vi "Calculate Bit Error Ratio.vi"(0 "in DFE mode?":bool, 5 "positive counts":T1, 7 "negative counts":T1, 11 "error in":errorcluster) -> (4 "bit error ratio":dbl, 6 "sample count":u64, 8 "error count":u64, 15 "error out":errorcluster)   [LabVIEW 2015, in "niHighSpeedSerial Eye Scan Single Point v1 Host.lvclass"]
doc: "Calculates the Bit Error Rate.\nWhen in LPM mode, the BER rate is computed as the (error count + 1)/(sample count)\nWhen in DFE mode, the BER rate is computed by taking the average of the positive BER and negative BER.\n\n<B>Input Parameters</B>\n\n<B>in DFE mode?</B> is true if Eye Scan is configured for DFE Equalization Mode.\n\n<B>positive counts</B> contains the positive UT sign sample and error counts when using DFE Equalization Mode.\nWhen using LPM Equalization Mode, contains the sample and error counts.\n\n<B>positive counts.sample count</B> is the positive sample count when using DFE mode, or the entire sample count when using LPM mode.\n\n<B>positive counts.error count</B> is the positive error count when using DFE mode, or the entire error count when using LPM mode.\n\n<B>negative counts</B> contains the negative UT sign sample and error counts when using DFE Equalization Mode.\nWhen using LPM Equalization Mode, 'negative counts' is unused.\n\n<B>negative counts.sample count</B> is the negative sample count when using DFE mode, or unused when using LPM mode.\n\n<B>negative counts.error count</B> is the negative error count when using DFE mode, or unused when using LPM mode.\n\n<B>error in</B> describes error conditions that occur before this node runs. This input provides standard 'error in' functionality.\n\n<B>Output Parameters</B>\n\n<B>bit error rate</B> is the calculated statistical bit error rate based on the number of error counts and sample counts received.\n\n<B>sample count</B> is the number of samples that have been measured on this point.\n\n<B>error count</B> is the number of errors that have been measured on this point.\n\n<B>error out</B> contains error information. This output provides standard 'error out' functionality."
uses:
  <instrlib>/niHighSpeedSerial/Eye Scan/v1/Host/Impl/Single Point/niHighSpeedSerial Eye Scan Single Point v1 Host.lvclass
  <instrlib>/niHighSpeedSerial/Eye Scan/v1/Host/Impl/Single Point/Private/Counts.ctl
  <instrlib>/niHighSpeedSerial/Eye Scan/v1/Host/Common/niHighSpeedSerial Eye Scan Common v1 Host.lvlib
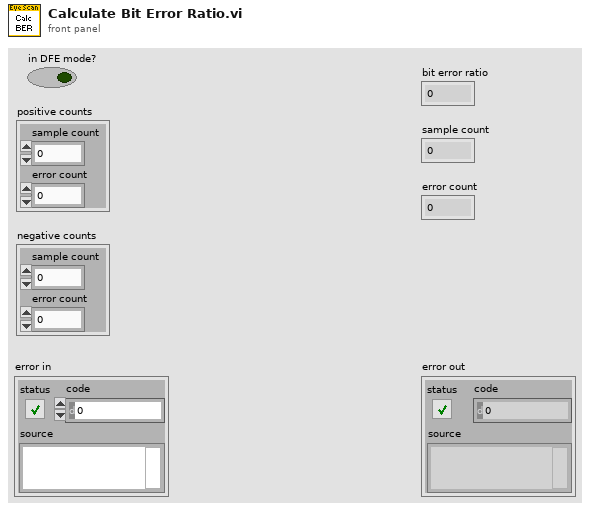
[diagram p1: front panel]
types:
  T1 = typedef "niHighSpeedSerial Eye Scan Single Point v1 Host.lvclass/Counts.ctl" = cluster{"sample count":u64, "error count":u16}
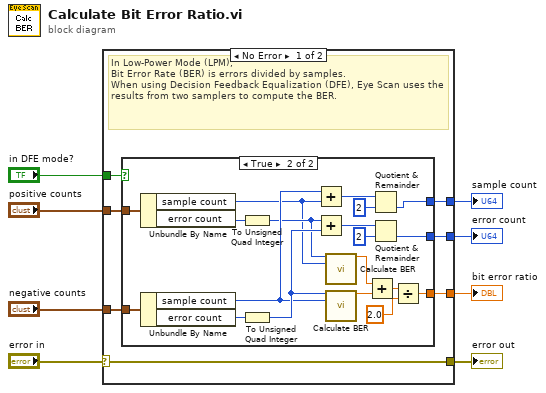
[diagram p0: block diagram]
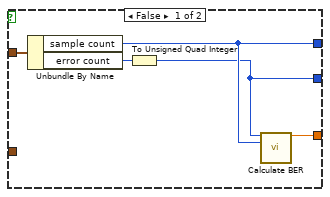
[diagram p2: hidden frame]
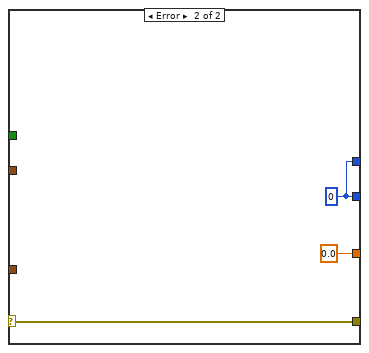
[diagram p3: hidden frame]
diagram:
  n1 = case shown="No Error" "error in" {
    selector: "error in" -> [w9 w42]
    tunnel: [w15 0.0] -> w8
    tunnel: [w14 w41] -> w7
    tunnel: [w13 w41] -> w6
    tunnel: "negative counts" -> [w12 _]
    tunnel: "positive counts" -> [w11 _]
    tunnel: "in DFE mode?" -> [w10 _]
    tunnel: [w9 w42] -> w1
    frame No Error {
      # "In Low-Power Mode (LPM),\nBit Error Rate (BER) is errors divided by samples.\nWhen using Decision Feedback Equalization (DFE), Eye Scan uses the results from two samplers to compute the BER."
      n2 = case shown="True" w10 {
        tunnel: w11 -> [w20 w39]
        tunnel: w12 -> [_ w38]
        tunnel: [w17 w30] -> w13
        tunnel: [w16 w27] -> w14
        tunnel: [w18 w33] -> w15
        frame False {
          n3 = Unbundle By Name(w20) -> ("sample count"=w17:u64, "error count"=w19:u16)
          n4 = To Unsigned Quad Integer(1:w19) -> (0:w16:u64)
          n5 = call <instrlib>:"Calculate BER.vi"("error count"=w16, "sample count"=w17) -> ("BER"=w18:dbl)  [unwired: 13 in]
        }
        frame True {
          n6 = Unbundle By Name(w39) -> ("sample count"=w21:u64, "error count"=w37:u16)
          n7 = Unbundle By Name(w38) -> ("sample count"=w23:u64, "error count"=w36:u16)
          n8 = To Unsigned Quad Integer(1:w37) -> (0:w22:u64)
          n9 = To Unsigned Quad Integer(1:w36) -> (0:w24:u64)
          n10 = Add(x=w23, y=w21) -> (x+y=w31:u64)
          n11 = Add(x=w22, y=w24) -> (x+y=w28:u64)
          n12 = call <instrlib>:"Calculate BER.vi"("error count"=w22, "sample count"=w21) -> ("BER"=w26:dbl)  [unwired: 13 in]
          n13 = call <instrlib>:"Calculate BER.vi"("error count"=w24, "sample count"=w23) -> ("BER"=w25:dbl)  [unwired: 13 in]
          n14 = Add(x=w26, y=w25) -> (x+y=w35:dbl)
          n15 = Quotient & Remainder(x=w31, y=u64 2) -> (floor(x/y)=w30:u64)  [unwired: 1 out]
          n16 = Quotient & Remainder(x=w28, y=u64 2) -> (floor(x/y)=w27:u64)  [unwired: 1 out]
          n17 = Divide(x=w35, y=2.0) -> (x/y=w33:dbl)
        }
      }
    }
    frame Error {
      w41 = u64 0
    }
  }
  "bit error ratio" <- w8
  "error count" <- w7
  "sample count" <- w6
  "error out" <- w1
